vi "20151030 Kalman filter module.vi"(7 "Action":enum16{"initialize", "update"}(ring)=enum."update", 8 "error in":errorcluster, 9 "Looptime":u32, 10 "newAngle":dbl format="%#_13g", 11 "newRate":dbl format="%#_13g") -> (0 "error out":errorcluster, 3 "x_angle":dbl)   [LabVIEW 2013]
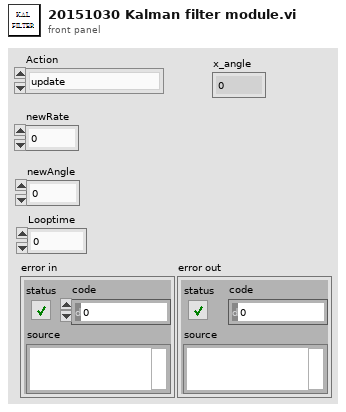
[diagram p1: front panel]
types:
  T1 = cluster{"P_00":dbl, "P_01":dbl, "P_10":dbl, "P_11":dbl, "x_bias":dbl}
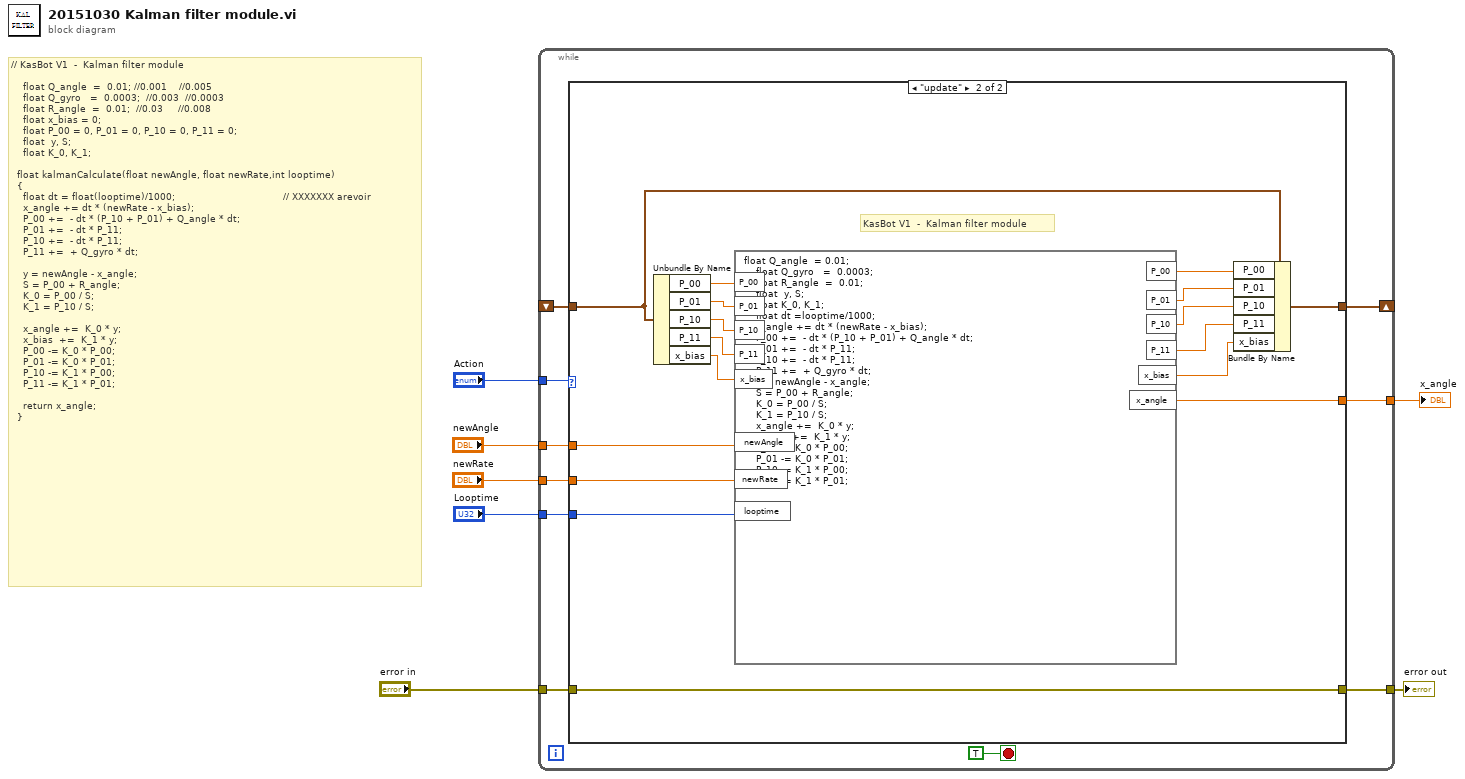
[diagram p0: block diagram]
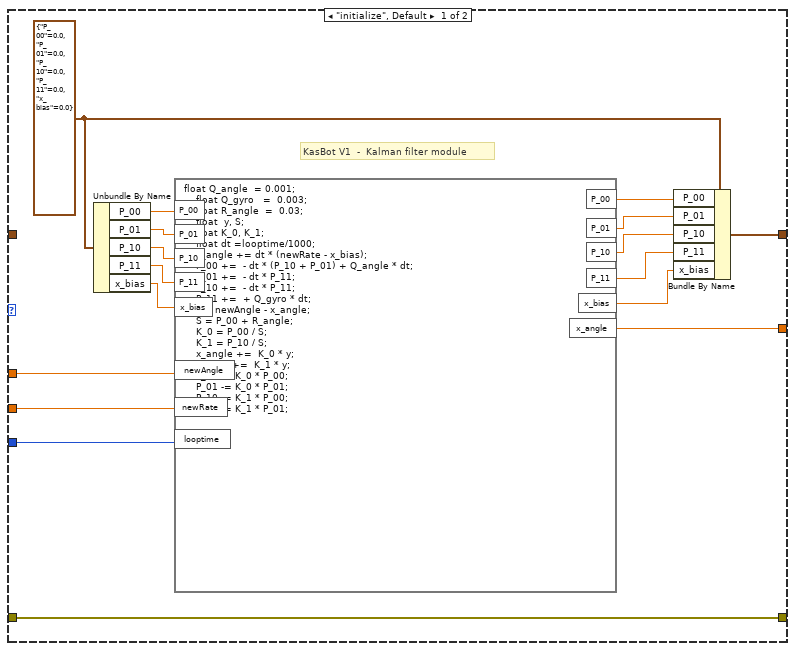
[diagram p2: hidden frame]
diagram:
  # "// KasBot V1  -  Kalman filter module\n\n    float Q_angle  =  0.01; //0.001    //0.005\n    float Q_gyro   =  0.0003;  //0.003  //0.0003\n    float R_angle  =  0.01;  //0.03     //0.008\n    float x_bias = 0;\n    float P_00 = 0, P_01 = 0, P_10 = 0, P_11 = 0;\t\n    float  y, S;\n    float K_0, K_1;\n\n  float kalmanCalculate(float newAngle, float newRate,int looptime)\n  {\n    float dt = float(looptime)/1000;                                    // XXXXXXX arevoir\n    x_angle += dt * (newRate - x_bias);\n    P_00 +=  - dt * (P_10 + P_01) + Q_angle * dt;\n    P_01 +=  - dt * P_11;\n    P_10 +=  - dt * P_11;\n    P_11 +=  + Q_gyro * dt;\n    \n    y = newAngle - x_angle;\n    S = P_00 + R_angle;\n    K_0 = P_00 / S;\n    K_1 = P_10 / S;\n    \n    x_angle +=  K_0 * y;\n    x_bias  +=  K_1 * y;\n    P_00 -= K_0 * P_00;\n    P_01 -= K_0 * P_01;\n    P_10 -= K_1 * P_00;\n    P_11 -= K_1 * P_01;\n    \n    return x_angle;\n  }"
  n1 = while {
    shift-right: [w11] -> _
    shift-left: _ -> [w15]
    tunnel: "Action" -> [w16]
    tunnel: "Looptime" -> [w14]
    tunnel: "newAngle" -> [w13]
    tunnel: "newRate" -> [w12]
    tunnel: [w10] -> w3
    tunnel: "error in" -> [w9]
    tunnel: [w8] -> w1
    stop <- TRUE stop-if-true
    n2 = case shown="\"update\"" w16 {
      tunnel: w15 -> [_ w37]
      tunnel: w14 -> [w32 w49]
      tunnel: w13 -> [w34 w51]
      tunnel: w12 -> [w33 w50]
      tunnel: [w20 w38] -> w11
      tunnel: [w19 w36] -> w10
      tunnel: w9 -> [w18 w35]
      tunnel: [w18 w35] -> w8
      frame "initialize", Default {
        w26 = T1 {"P_00"=0.0, "P_01"=0.0, "P_10"=0.0, "P_11"=0.0, "x_bias"=0.0}
        # "KasBot V1  -  Kalman filter module"
        n3 = Unbundle By Name(w26) -> ("P_00"=w31:dbl, "P_01"=w30:dbl, "P_10"=w29:dbl, "P_11"=w28:dbl, "x_bias"=w27:dbl)
        n4 = formula code="float Q_angle  = 0.001;\n    float Q_gyro   =  0.003;\n    float R_angle  =  0.03;\n    float  y, S;\n    float K_0, K_1;\n    float dt =looptime/1000; \n    x_angle += dt * (newRate - x_bias);\n    P_00 +=  - dt * (P_10 + P_01) + Q_angle * dt;\n    P_01 +=  - dt * P_11;\n    P_10 +=  - dt * P_11;\n    P_11 +=  + Q_gyro * dt;\n    y = newAngle - x_angle;\n    S = P_00 + R_angle;\n    K_0 = P_00 / S;\n    K_1 = P_10 / S;\n    x_angle +=  K_0 * y;\n    x_bias  +=  K_1 * y;\n    P_00 -= K_0 * P_00;\n    P_01 -= K_0 * P_01;\n    P_10 -= K_1 * P_00;\n    P_11 -= K_1 * P_01;"("looptime"=w32, "newAngle"=w34, "newRate"=w33, "P_00"=w31, "P_01"=w30, "P_10"=w29, "P_11"=w28, "x_bias"=w27) -> ("x_angle"=w19:dbl, "P_00"=w25:dbl, "P_01"=w24:dbl, "P_11"=w22:dbl, "P_10"=w23:dbl, "x_bias"=w21:dbl)
        n5 = Bundle By Name(cluster=w26, "P_00"=w25, "P_01"=w24, "P_10"=w23, "P_11"=w22, "x_bias"=w21) -> (w20:T1)
      }
      frame "update" {
        # "KasBot V1  -  Kalman filter module"
        n6 = Unbundle By Name(w37) -> ("P_00"=w48:dbl, "P_01"=w47:dbl, "P_10"=w46:dbl, "P_11"=w45:dbl, "x_bias"=w44:dbl)
        n7 = formula code="float Q_angle  = 0.01;\n    float Q_gyro   =  0.0003;\n    float R_angle  =  0.01;\n    float  y, S;\n    float K_0, K_1;\n    float dt =looptime/1000; \n    x_angle += dt * (newRate - x_bias);\n    P_00 +=  - dt * (P_10 + P_01) + Q_angle * dt;\n    P_01 +=  - dt * P_11;\n    P_10 +=  - dt * P_11;\n    P_11 +=  + Q_gyro * dt;\n    y = newAngle - x_angle;\n    S = P_00 + R_angle;\n    K_0 = P_00 / S;\n    K_1 = P_10 / S;\n    x_angle +=  K_0 * y;\n    x_bias  +=  K_1 * y;\n    P_00 -= K_0 * P_00;\n    P_01 -= K_0 * P_01;\n    P_10 -= K_1 * P_00;\n    P_11 -= K_1 * P_01;"("looptime"=w49, "newAngle"=w51, "newRate"=w50, "P_00"=w48, "P_01"=w47, "P_10"=w46, "P_11"=w45, "x_bias"=w44) -> ("x_angle"=w36:dbl, "P_00"=w43:dbl, "P_01"=w42:dbl, "P_11"=w40:dbl, "P_10"=w41:dbl, "x_bias"=w39:dbl)
        n8 = Bundle By Name(cluster=w37, "P_00"=w43, "P_01"=w42, "P_10"=w41, "P_11"=w40, "x_bias"=w39) -> (w38:T1)
      }
    }
  }
  "x_angle" <- w3
  "error out" <- w1
